vi "Parse Results.vi"(1 "measurement line":string) -> (8 "measurement results":T1)   [LabVIEW 2019, in "Andeen-Hagerling 2700A.lvlib"]
doc: "Parses a line of measurement results. The output is a cluster consisting of the error code, frequency, capacitance, loss, greater than flag, and voltage."
uses:
  Andeen-Hagerling 2700A.lvlib
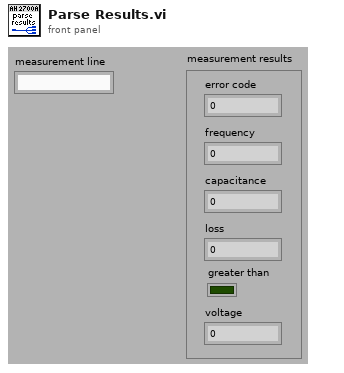
[diagram p1: front panel]
types:
  T1 = cluster{"error code":i32, "frequency":dbl, "capacitance":dbl, "loss":dbl, "greater than":bool, "voltage":dbl}
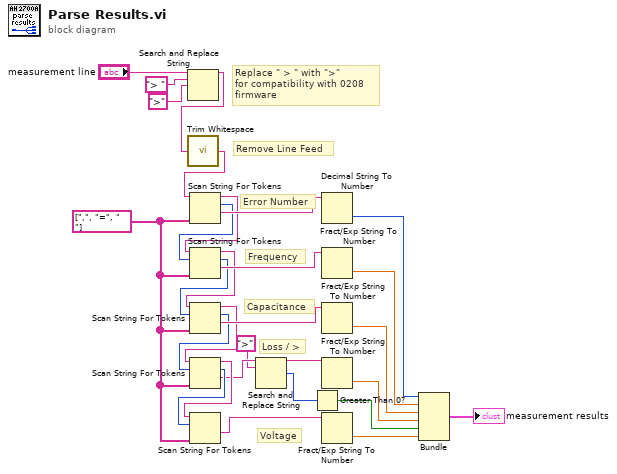
[diagram p0: block diagram]
diagram:
  w25 = string[] [",", "=", " "] ("delimiters (\\s,\\t,\\r,\\n)")
  # "Remove Line Feed"
  # "Loss / >"
  # "Voltage"
  # "Capacitance"
  # "Frequency"
  # "Error Number"
  # "Replace \" > \" with \">\"\nfor compatibility with 0208\nfirmware"
  n1 = Search and Replace String(input string="measurement line", search string="> ", replace string=">" ("replace string (\"\")")) -> (result string=w4:string)  [unwired: 5 in, 3 out]
  n2 = call <vilib>:"Trim Whitespace.vi"("string"=w4) -> ("trimmed string"=w3:string)  [unwired: 1 in]
  n3 = Scan String For Tokens(6:w25, 9:w3) -> (1:w26:string, 2:w21:i32, 3:w17:string)  [unwired: 4 in, 1 out]
  n4 = Scan String For Tokens(6:w25, 8:w21, 9:w17) -> (1:w27:string, 2:w22:i32, 3:w18:string)  [unwired: 3 in, 1 out]
  n5 = Scan String For Tokens(6:w25, 8:w22, 9:w18) -> (1:w28:string, 2:w23:i32, 3:w19:string)  [unwired: 3 in, 1 out]
  n6 = Scan String For Tokens(6:w25, 8:w23, 9:w19) -> (1:w10:string, 2:w24:i32, 3:w20:string)  [unwired: 3 in, 1 out]
  n7 = Scan String For Tokens(6:w25, 8:w24, 9:w20) -> (1:w29:string)  [unwired: 3 in, 3 out]
  n8 = Search and Replace String(input string=w10, search string=">" ("regular expression")) -> (result string=w8:string, number of replacements=w2:i32)  [unwired: 6 in, 2 out]
  n9 = Greater Than 0?(x=w2) -> (x > 0?=w1:bool)
  n10 = Decimal String To Number(string=w26) -> (number=w12:i32)  [unwired: 2 in, 1 out]
  n11 = Fract/Exp String To Number(string=w27) -> (number=w13:dbl)  [unwired: 3 in, 1 out]
  n12 = Fract/Exp String To Number(string=w28) -> (number=w14:dbl)  [unwired: 3 in, 1 out]
  n13 = Fract/Exp String To Number(string=w8) -> (number=w15:dbl)  [unwired: 3 in, 1 out]
  n14 = Fract/Exp String To Number(string=w29) -> (number=w16:dbl)  [unwired: 3 in, 1 out]
  n15 = Bundle(w12, w13, w14, w15, w1, w16) -> (→"measurement results":cluster{i32, dbl, dbl, dbl, bool, dbl})  [unwired: 1 in]
